vi "Digital Out Test_TS.vi"(10 "Message IN":string) -> (0 "error out":errorcluster, 1 "Result (bool)":bool, 2 "Message OUT":string, 3 "VISA resource name 2":refnum<visa-resource-name>)   [LabVIEW 2022 SP3]
uses:
  <vilib>/DAQmx/read.llb/DAQmx Read (Digital 1D Bool NChan 1Samp 1Line).vi
  <vilib>/DAQmx/miscellaneous.llb/DAQmx Fill In Error Info.vi
panel:
  in  "error IO":errorcluster
  out "Result (color)":u32(colorbox)
  out "cDAQ DI Reading":bool[](array[boolean])
  out "LC DO Cmd":bool[](array[boolean])
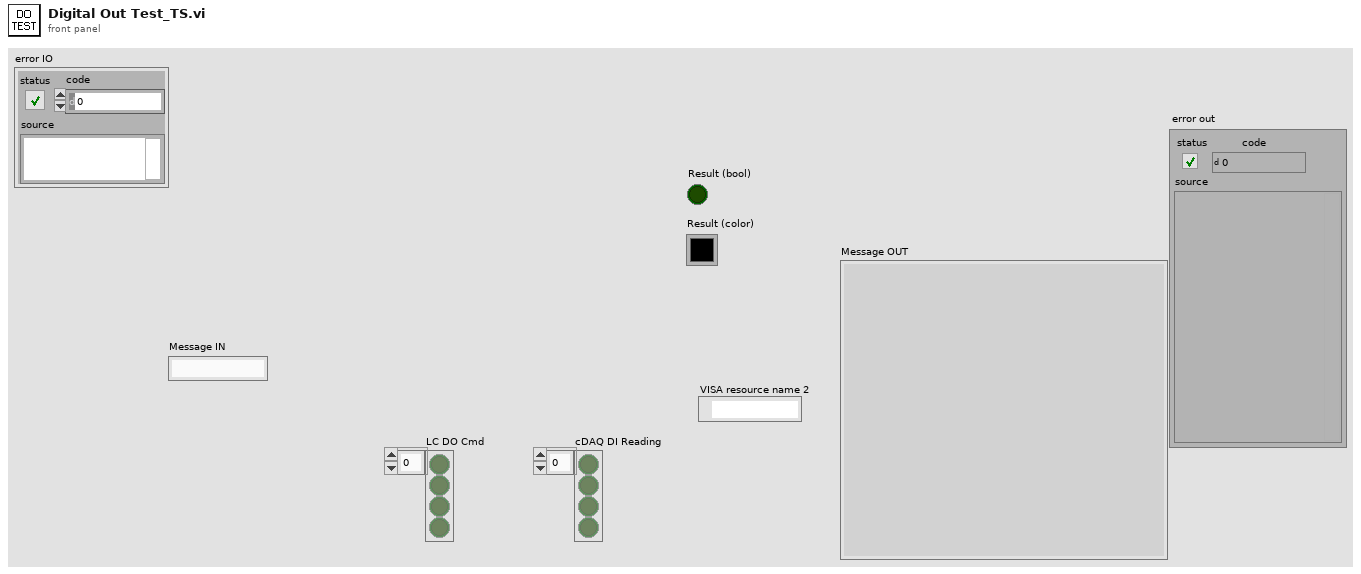
[diagram p1: front panel]
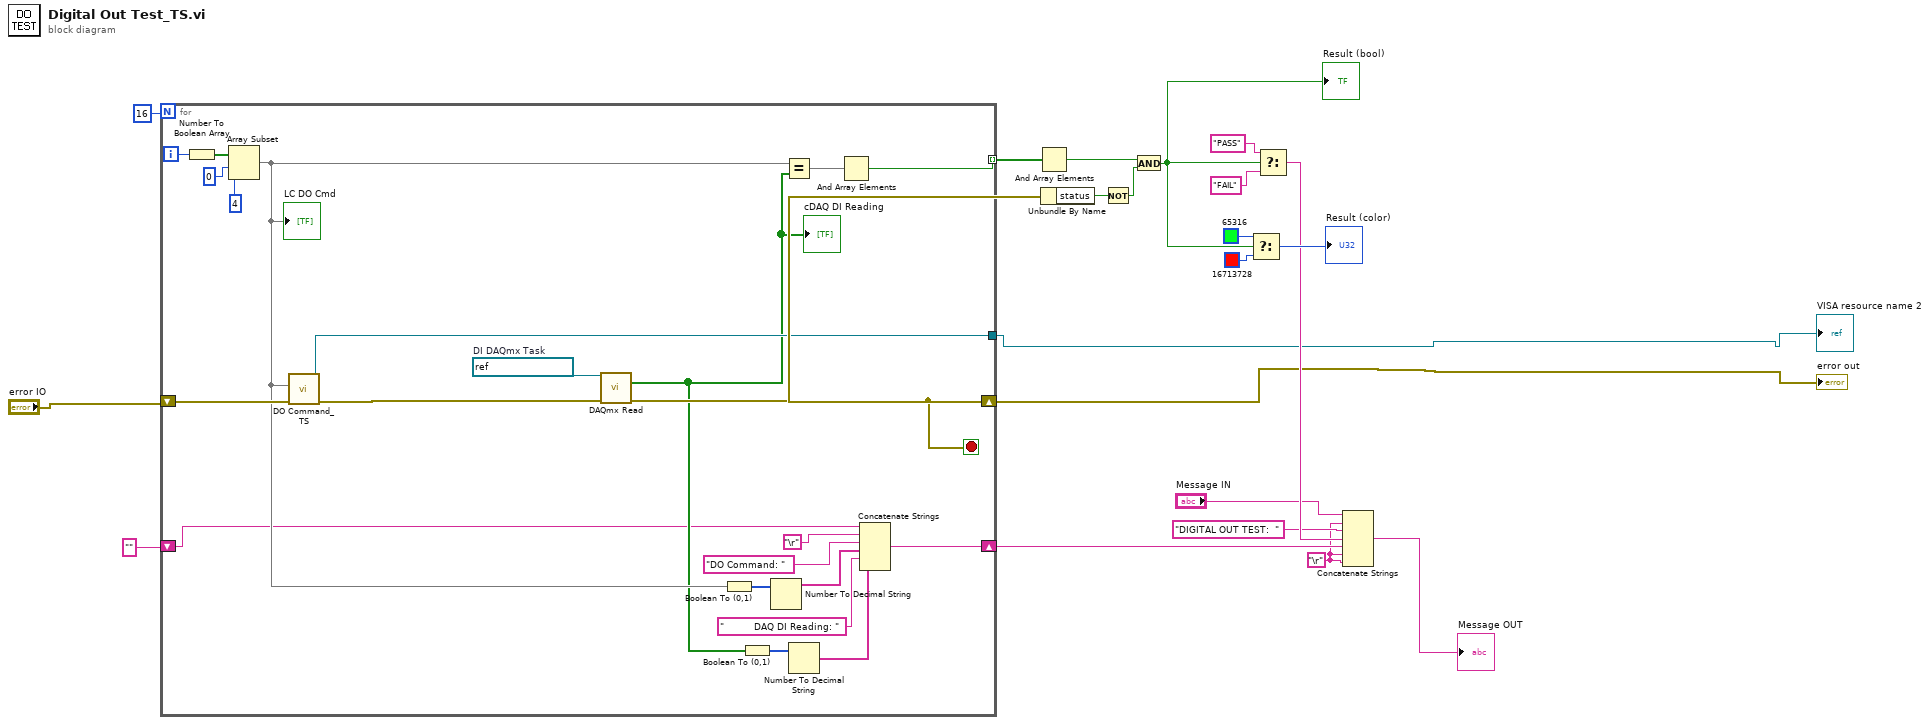
[diagram p0: block diagram]
diagram:
  w5 = "\r"
  n1 = for {
    N: 16 -> [_]
    shift-right: [w38] -> w2
    shift-left: "error IO" -> [w41]
    tunnel: [w40] -> w1
    tunnel: [w43] -> w21 mode=indexing
    shift-right: [w25] -> w10
    shift-left: "" -> [w24]
    i -> [w23]
    stop <- w38 stop-if-true
    w39 = refnum<k21> "FTS2_DigitalIn"  # DI DAQmx Task
    n2 = Number To Boolean Array(number=w23) -> (Boolean array=w35:bool[])
    n3 = Array Subset(array=w35, index=0, length=4) -> (w27:bool[])
    "LC DO Cmd" <- w27
    n4 = call "DO Command_TS.vi"("error in (no error)"=w41, "DO Command"=w27) -> ("error out"=w22:errorcluster, "VISA Refnum out"=w40:refnum<visa-resource-name>)  [unwired: 8 in]
    n5 = call-poly <vilib>:"DAQmx Read.vi"("task/channels in"=w39, "error in"=w22) -> ("data"=w26:bool[], "error out"=w38:errorcluster)  [unwired: 11 in, 1 out]
    "cDAQ DI Reading" <- w26
    n6 = Boolean To (0,1)(Boolean=w27) -> (0, 1=w29:i16[])
    n7 = Boolean To (0,1)(Boolean=w26) -> (0, 1=w28:i16[])
    n8 = Number To Decimal String(number=w29) -> (decimal integer string=w32:string[])  [unwired: 1 in]
    n9 = Equal?(x=w27, y=w26) -> (x = y?=w42:bool[])
    n10 = Number To Decimal String(number=w28) -> (decimal integer string=w34:string[])  [unwired: 1 in]
    n11 = And Array Elements(Boolean array=w42) -> (logical AND=w43:bool)
    n12 = Concatenate Strings(w24, "\r", "DO Command: ", w32, "          DAQ DI Reading: ", w34) -> (w25:string)
  }
  "VISA resource name 2" <- w1
  "error out" <- w2
  n13 = And Array Elements(Boolean array=w21) -> (logical AND=w11:bool)
  n14 = Unbundle By Name(w2) -> ("status"=w14:bool)
  n15 = Not(x=w14) -> (.not. x?=w13:bool)
  n16 = And(x=w11, y=w13) -> (x .and. y?=w12:bool)
  "Result (bool)" <- w12
  n17 = Select(t=u32 65316 ("Result (color)"), s=w12, f=u32 16713728 ("Result (color)")) -> (s? t:f=→"Result (color)":u32)
  n18 = Select(t="PASS", s=w12, f="FAIL") -> (s? t:f=w8:string)
  n19 = Concatenate Strings("Message IN", w5, "DIGITAL OUT TEST:  ", w8, w10, w5, w5) -> (→"Message OUT":string)
